vi "Actor Core.vi"(8 "error in":errorcluster caption="错误输入", 11 "HTTP发送 in":refnum<class "HTTP发送.lvclass"> caption="操作者输入") -> (0 "error out":errorcluster caption="错误输出", 3 "Actor out":refnum<class "Actor.lvclass"> caption="操作者输出")   [LabVIEW 2022 SP3, in "工况数据上传.lvlib" / "HTTP发送.lvclass"]
doc: "(<B>Filename</B>: Actor Framework.lvlib:Actor.lvclass:Actor Core.vi)\n\nReceives messages to the actor, reacts to them, and initiates any error handling that may shut the actor down.\n\nDescendant classes may override this VI to append parallel tasks for the actor to complete while it handles messages.使用调用父方法节点实现重写。"
uses:
  C:/Program Files (x86)/National Instruments/LabVIEW 2022/vi.lib/ActorFramework/Actor/Actor.lvclass
  <vilib>/ActorFramework/Actor/Actor.lvclass
  <vilib>/ActorFramework/Actor/Actor.lvclass/Actor.ctl
  <vilib>/ActorFramework/Message Enqueuer/Message Enqueuer.lvclass/Message Enqueuer.ctl
  <vilib>/ActorFramework/Message Enqueuer/Init from Existing Queue.vi
  <vilib>/ActorFramework/Message Enqueuer/Enqueue.vi
  C:/Program Files (x86)/National Instruments/LabVIEW 2022/vi.lib/ActorFramework/Message/Message.lvclass
  <vilib>/ActorFramework/Stop Msg/Stop Msg.lvclass
  <vilib>/ActorFramework/Message Priority Queue/Priority Enqueue.vi
  <vilib>/ActorFramework/Message Enqueuer/Message Enqueuer.lvclass
panel:
  in  "停止按钮":bool
  in  "response":T1
  in  "json":string[](array[string])
  in  "配置":T2
  out "JSON字符串":string
  out "time":string="2021-05-08 14:02:02"
  out "body":string caption="体部"
  out "headers":string caption="头部"
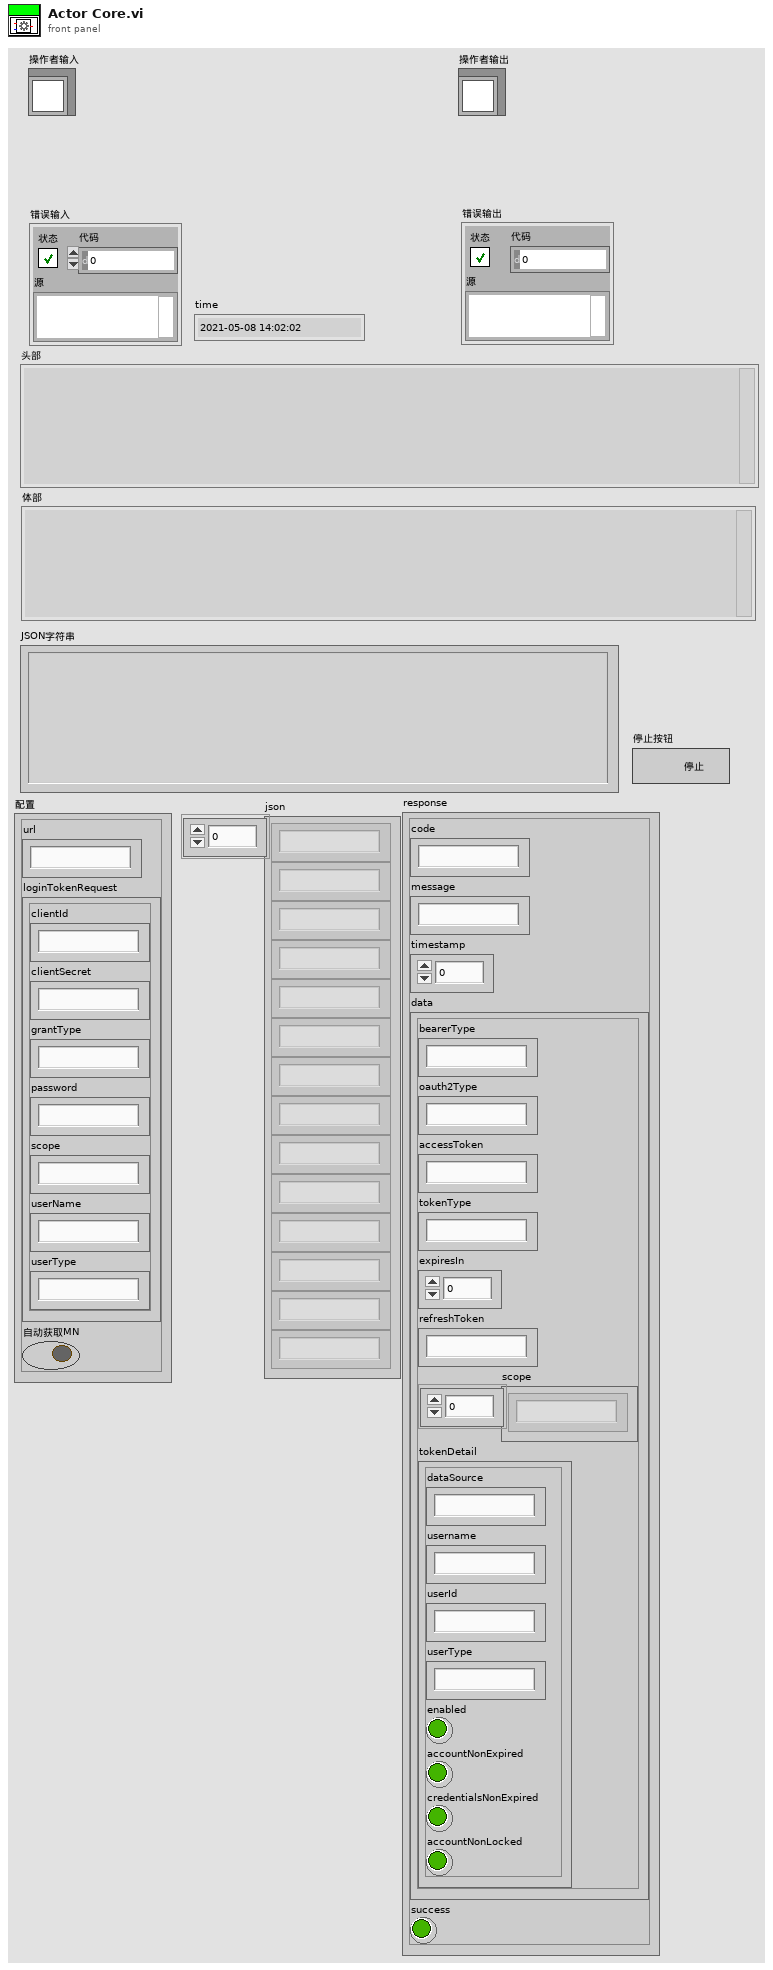
[diagram p1: front panel]
types:
  T1 = cluster{"code":string, "message":string, "timestamp":u64, "data":cluster{"bearerType":string, "oauth2Type":string, "accessToken":string, "tokenType":string, "expiresIn":u64, "refreshToken":string, "scope":string[], "tokenDetail":cluster{"dataSource":string, "username":string, "userId":string, "userType":string, "enabled":bool, "accountNonExpired":bool, "credentialsNonExpired":bool, "accountNonLocked":bool}}, "success":bool}
  T2 = cluster{"url":string, "loginTokenRequest":cluster{"clientId":string, "clientSecret":string, "grantType":string, "password":string, "scope":string, "userName":string, "userType":string}, "自动获取MN":bool}
  T3 = enum32{"Invalid", "Standard", "Closed", "Hidden", "Minimized", "Maximized"}
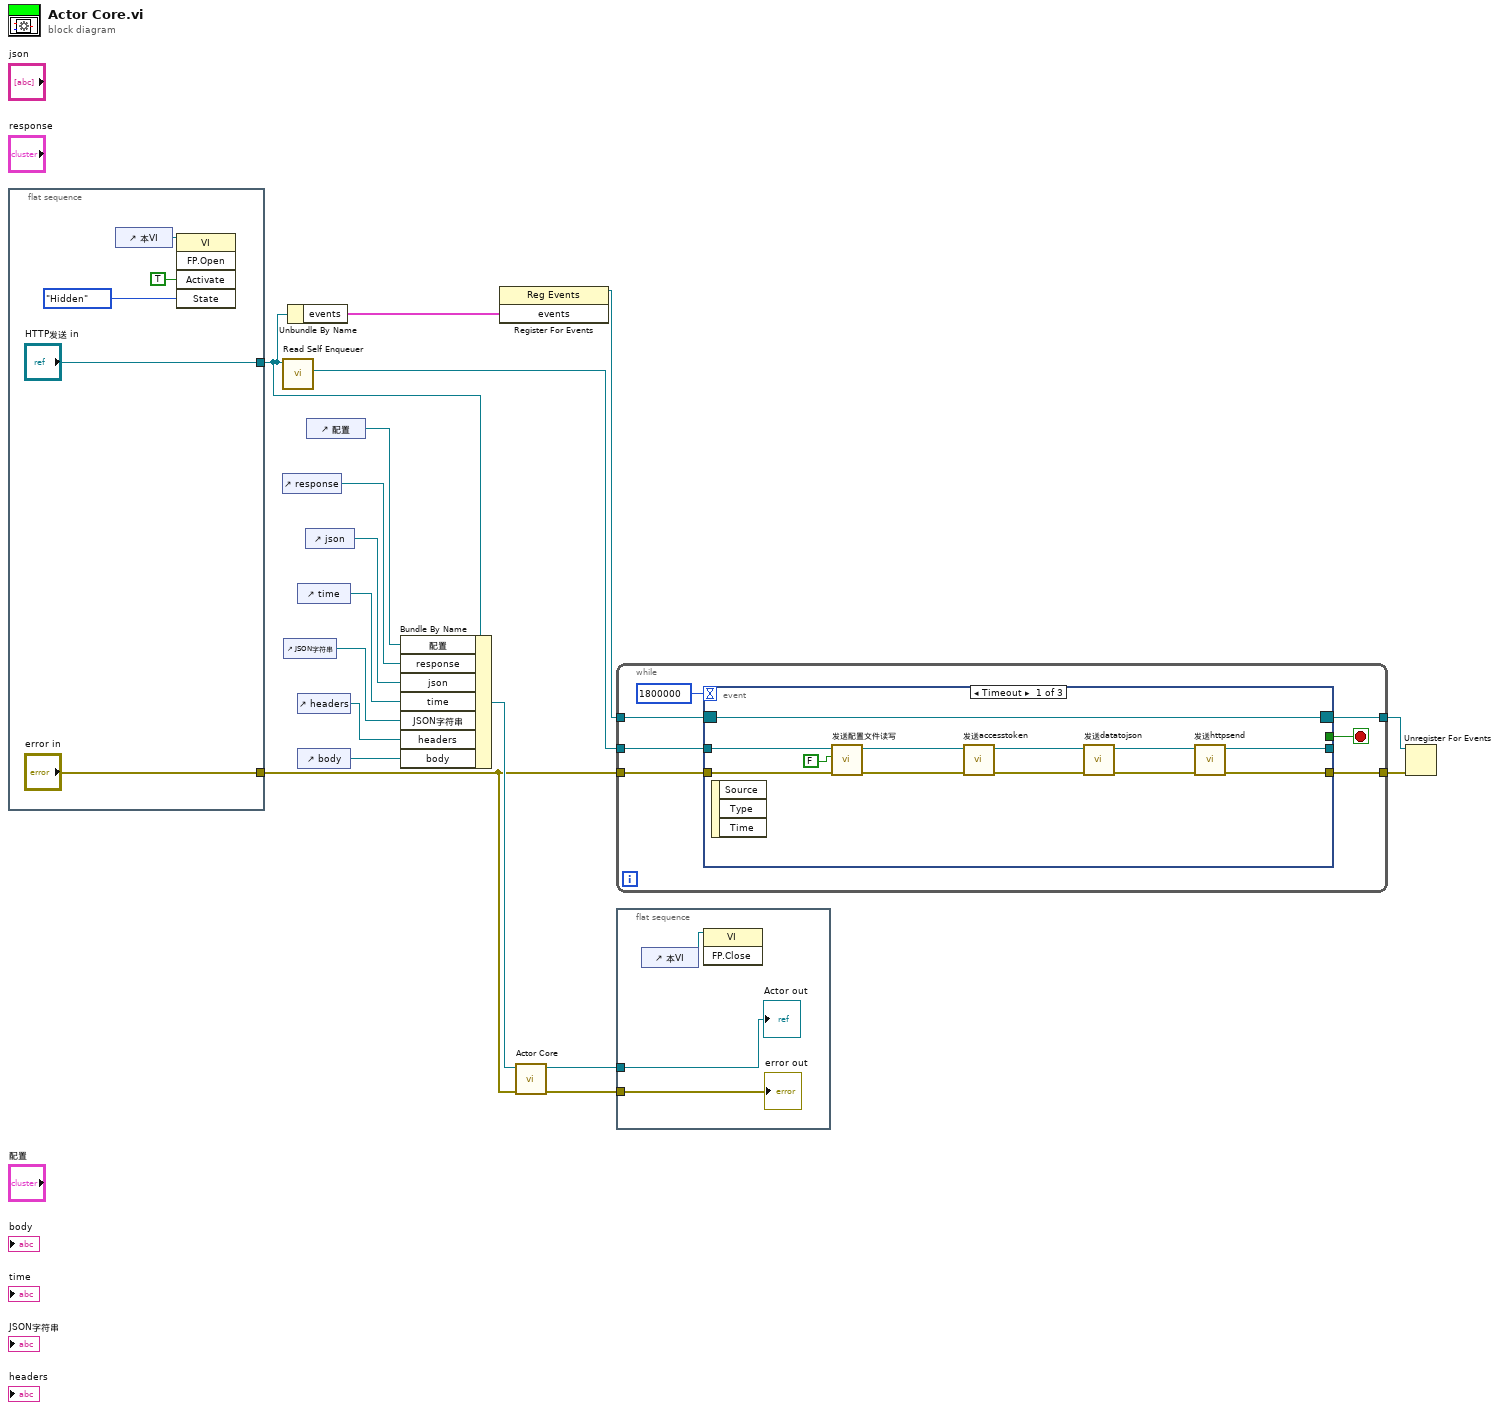
[diagram p0: block diagram]
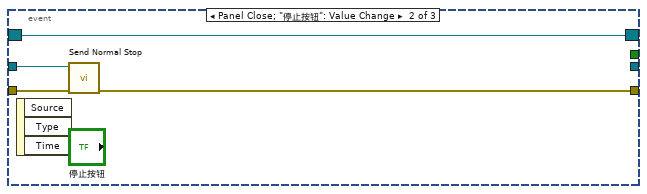
[diagram p2: hidden frame]
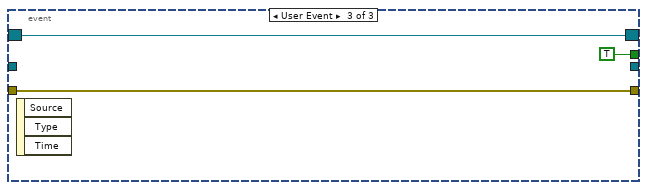
[diagram p3: hidden frame]
diagram:
  n1 = flat-sequence {
    tunnel: ["error in"] -> w6
    tunnel: ["HTTP发送 in"] -> w5
    frame #0 {
      n2 = control-ref of="本VI"() -> (w18:refnum<vi>)
      n3 = invoke class="VI" method="FP.Open"(reference=w18, "Activate"=TRUE ("激活？"), "State"=T3."Hidden" ("状态")) -> ()  [unwired: 2 in, 5 out]
    }
  }
  n4 = call <vilib>:"Read Self Enqueuer.vi"("Actor"=w5) -> ("Self Enqueuer"=w7:refnum<class "Message Enqueuer.lvclass">)  [unwired: 10 in]
  n5 = control-ref of="response"() -> (w15:refnum<vi>)
  n6 = control-ref of="JSON字符串"() -> (w12:refnum<vi>)
  n7 = Unbundle By Name(w5) -> ("events"=w4:cluster{"Stop":refnum<user-event>})
  n8 = control-ref of="time"() -> (w11:refnum<vi>)
  n9 = control-ref of="headers"() -> (w10:refnum<vi>)
  n10 = control-ref of="body"() -> (w9:refnum<vi>)
  n11 = control-ref of="json"() -> (w14:refnum<vi>)
  n12 = control-ref of="配置"() -> (w13:refnum<vi>)
  n13 = Bundle By Name(cluster=w5, "配置"=w13, "response"=w15, "json"=w14, "time"=w11, "JSON字符串"=w12, "headers"=w10, "body"=w9) -> (w8:refnum<class "HTTP发送.lvclass">)
  n14 = register-events(w4) -> (reference out=w3:refnum<event-registration>)  [unwired: 2 in, 1 out]
  n15 = call-parent "Actor Core.vi"("error in"=w6, "Actor in"=w8) -> ("error out"=w17:errorcluster, "Actor out"=w16:refnum<class "Actor.lvclass">)  [unwired: 8 in]
  n16 = while {
    tunnel: w7 -> [w29]
    tunnel: w6 -> [w28]
    tunnel: w3 -> [w25]
    tunnel: [w24] -> w2
    tunnel: [w23] -> w1
    stop <- w26 stop-if-true
    n17 = event shown="[0] Timeout" {
      selector: w25 -> [w30 w42 w46]
      dyn-events: [w30 w42 w46] -> w24
      timeout: u32 1800000 ("等待时间（毫秒）") -> [_ _ _]
      tunnel: w29 -> [w39 w45 _]
      tunnel: w28 -> [w37 w44 w47]
      tunnel: [w33 _ _] -> _
      tunnel: [w31 w43 w47] -> w23
      tunnel: [_ _ TRUE] -> w26
      event Timeout {
        n18 = event-data() -> ()  [unwired: 1 in, 3 out]
        n19 = call "发送配置文件读写.vi"("error in (no error)"=w37, "write?"=FALSE, "Message Enqueuer"=w39) -> ("error out"=w35:errorcluster, "Message Enqueuer out"=w36:refnum<class "Message Enqueuer.lvclass">)  [unwired: 7 in]
        n20 = call "发送accesstoken.vi"("error in (no error)"=w35, "Message Enqueuer"=w36) -> ("error out"=w40:errorcluster, "Message Enqueuer out"=w41:refnum<class "Message Enqueuer.lvclass">)  [unwired: 8 in]
        n21 = call "发送datatojson.vi"("error in (no error)"=w40, "Message Enqueuer"=w41) -> ("error out"=w32:errorcluster, "Message Enqueuer out"=w34:refnum<class "Message Enqueuer.lvclass">)  [unwired: 8 in]
        n22 = call "发送httpsend.vi"("error in (no error)"=w32, "Message Enqueuer"=w34) -> ("error out"=w31:errorcluster, "Message Enqueuer out"=w33:refnum<class "Message Enqueuer.lvclass">)  [unwired: 8 in]
      }
      event Panel Close; "停止按钮": Value Change {
        n23 = event-data() -> ()  [unwired: 1 in, 3 out]
        n24 = call <vilib>:"Send Normal Stop.vi"("error in (no error)"=w44, "Message Enqueuer"=w45) -> ("error out"=w43:errorcluster)  [unwired: 9 in]
      }
      event User Event {
        n25 = event-data() -> ()  [unwired: 1 in, 3 out]
      }
    }
  }
  n26 = flat-sequence {
    tunnel: w17 -> [w50]
    tunnel: w16 -> [w51]
    frame #0 {
      n27 = control-ref of="本VI"() -> (w49:refnum<vi>)
      n28 = invoke class="VI" method="FP.Close"(reference=w49) -> ()  [unwired: 2 in, 3 out]
      "error out" <- w50
      "Actor out" <- w51
    }
  }
  n29 = Unregister For Events(event registration refnum=w2, error in=w1) -> ()  [unwired: 1 out]
